vi "disconnectCommand.vi"(8 "error in (no error)":errorcluster, 11 "MiddlewareSALThisComponent in":refnum<class "MiddlewareSALThisComponent.lvclass">) -> (0 "error out":errorcluster, 3 "MiddlewareSALThisComponent out":refnum<class "MiddlewareSALThisComponent.lvclass">)   [LabVIEW 2016, in "MiddlewareSALThisComponent.lvclass"]
uses:
  MiddlewareSALThisComponent.lvclass
  ComponentTemplateCore/ComponentModel/ComponentModel/MiddlewareSAL/MiddlewareSAL.lvclass
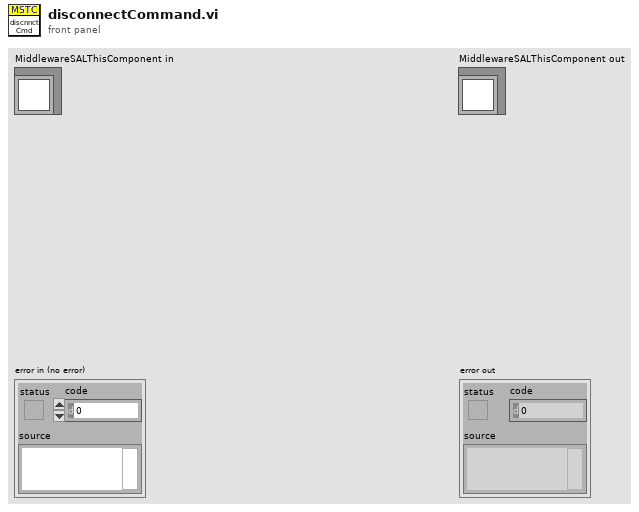
[diagram p1: front panel]
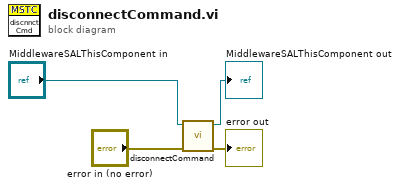
[diagram p0: block diagram]
diagram:
  n1 = call-parent "disconnectCommand.vi"("error in (no error)"="error in (no error)", "Middleware in"="MiddlewareSALThisComponent in") -> ("error out"=→"error out":errorcluster, "Middleware out"=→"MiddlewareSALThisComponent out":refnum<class "MiddlewareSALThisComponent.lvclass">)  [unwired: 8 in]
